vi "Pre Launch Init.vi"(11 "Iterator Actor in":refnum<class "Iterator Actor.lvclass">) -> (0 "error out":errorcluster, 3 "Iterator Actor out":refnum<class "Iterator Actor.lvclass">)   [LabVIEW 2020, in "Iterator Actor.lvlib" / "Iterator Actor.lvclass"]
doc: "(<B>Filename</B>: Actor Framework.lvlib:Actor.lvclass:Pre Launch Init.vi)\n\nDefines behavior that occurs after the Launch Nested Actor method is invoked but before the actor's Actor Core method begins running.\n\nBy default, this method does nothing. A descendant class may override it to define behavior."
uses:
  Iterator Actor.lvclass
  Iterator Actor Abstract Messages/Iterator Report Iterations End Msg/Iterator Report Iterations End Msg.lvclass
  Iterator Actor Abstract Messages/Iterator Reply Msg/Iterator Reply Msg.lvclass
  Iterator Settings.ctl
  Active Stop Conditions.ctl
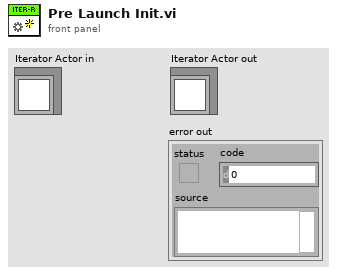
[diagram p1: front panel]
types:
  T1 = typedef "Iterator Actor.lvlib/Iterator Actor.lvclass/Iterator Settings.ctl" = cluster{"Prepare timeout (ms)":i32, "Iterate timeout (ms)":i32, "Conclude timeout (ms)":i32, "Iterate period (ms)":i32, "Number of iterations":i32, "Time before stop (ms)":i32, "Active Stop Conditions":T2, "Prepare Msg":refnum<class "Iterator Reply Msg.lvclass">, "Iterate Msg":refnum<class "Iterator Reply Msg.lvclass">, "Conclude Msg":refnum<class "Iterator Reply Msg.lvclass">, "Iterations End Report":refnum<class "Iterator Report Iterations End Msg.lvclass">}
  T2 = typedef "Iterator Actor.lvlib/Iterator Actor.lvclass/Active Stop Conditions.ctl" = cluster{"Number of Iterations":bool, "Time Elapsed":bool, "Iteration Result":bool}
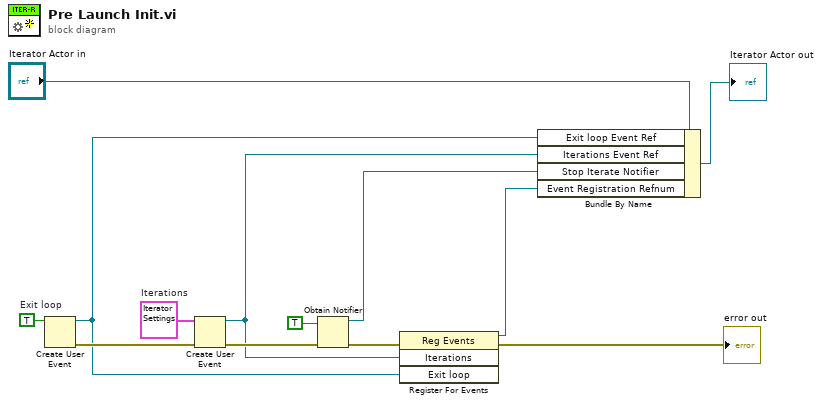
[diagram p0: block diagram]
diagram:
  w13 = T1 {"Prepare timeout (ms)"=0, "Iterate timeout (ms)"=0, "Conclude timeout (ms)"=0, "Iterate period (ms)"=0, "Number of iterations"=0, "Time before stop (ms)"=0, "Active Stop Conditions"={"Number of Iterations"=FALSE, "Time Elapsed"=FALSE, "Iteration Result"=FALSE}, "Prepare Msg"=refnum, "Iterate Msg"=refnum, "Conclude Msg"=refnum, "Iterations End Report"=refnum}  # Iterations
  w12 = TRUE  # Exit loop
  n1 = Create User Event(user event datatype=w12) -> (user event=w2:refnum<user-event>, error out=w4:errorcluster)  [unwired: 1 in]
  n2 = Create User Event(user event datatype=w13, error in=w4) -> (user event=w1:refnum<user-event>, error out=w3:errorcluster)
  n3 = Obtain Notifier(notification data type=TRUE, error in (no error)=w3) -> (notifier out=w10:refnum<notifier>, error out=w5:errorcluster)  [unwired: 2 in, 1 out]
  n4 = register-events(error in=w5, w1, w2) -> (reference out=w6:refnum<event-registration>, error out=→"error out":errorcluster)  [unwired: 1 in]
  n5 = Bundle By Name(cluster="Iterator Actor in", "Exit loop Event Ref"=w2, "Iterations Event Ref"=w1, "Stop Iterate Notifier"=w10, "Event Registration Refnum"=w6) -> (→"Iterator Actor out":refnum<class "Iterator Actor.lvclass">)
